vi "Write Waveform.vi"(8 "error in (no error)":errorcluster, 10 "Waveform":waveform(dbl), 11 "AOChData in":refnum<class "AOChData.lvclass">) -> (0 "error out":errorcluster, 3 "AOChData out":refnum<class "AOChData.lvclass">)   [LabVIEW 2015, in "Analog Output Channel.lvlib" / "AOChData.lvclass"]
uses:
  AOChData.lvclass
  AOChData.lvclass/AOChData.ctl
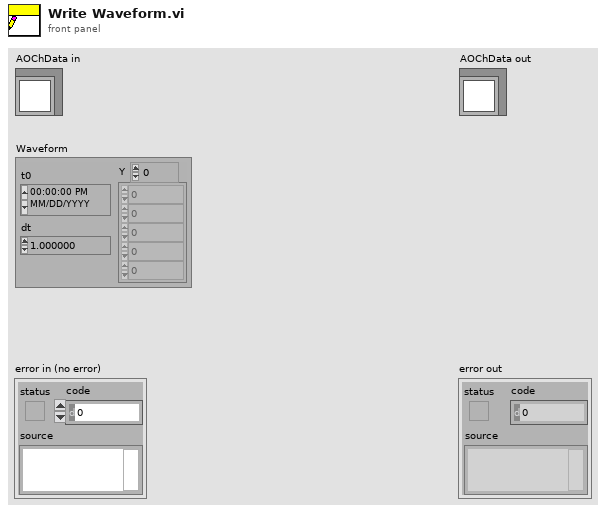
[diagram p1: front panel]
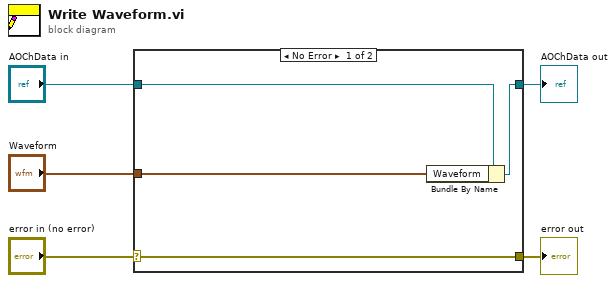
[diagram p0: block diagram]
diagram:
  n1 = case shown="No Error" "error in (no error)" {
    selector: "error in (no error)" -> [w9 w10]
    tunnel: [w9 w10] -> w4
    tunnel: [w7 w11] -> w2
    tunnel: "AOChData in" -> [w8 w11]
    tunnel: "Waveform" -> [w6 _]
    frame No Error {
      n2 = Bundle By Name(cluster=w8, "Waveform"=w6) -> (w7:refnum<class "AOChData.lvclass">)
    }
    frame Error {
    }
  }
  "error out" <- w4
  "AOChData out" <- w2
